vi "Generate Custom Trace.vi"(8 "error in (no error)":errorcluster, 10 "Custom Action":string) -> ()   [LabVIEW 2020, in "Actor Framework.lvlib"]
doc: "<p>Generates a DETT (Desktop Execution Trace Toolkit) User Generated Trace. The trace includes the source actor's ID (or debug alias, if available) and a custom message you define.</p>"
uses:
  Actor Framework.lvlib
  Support/Registration Mode.ctl
  Support/TDM Registration Mode.ctl
  Support/Localized Strings.vi
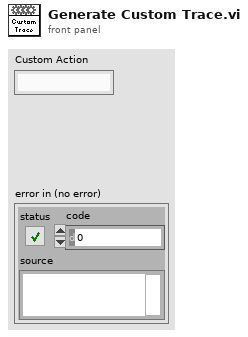
[diagram p1: front panel]
types:
  T1 = typedef "Actor Framework.lvlib/Registration Mode.ctl" = enum16{"Register Actor", "Get ID", "Get Enqueuer", "Deregister Actor", "Get Update Event", "Get All Actors"}
  T2 = typedef "Actor Framework.lvlib/TDM Registration Mode.ctl" = enum16{"Register TDM", "Get ID", "Get Notifier", "Deregister TDM"}
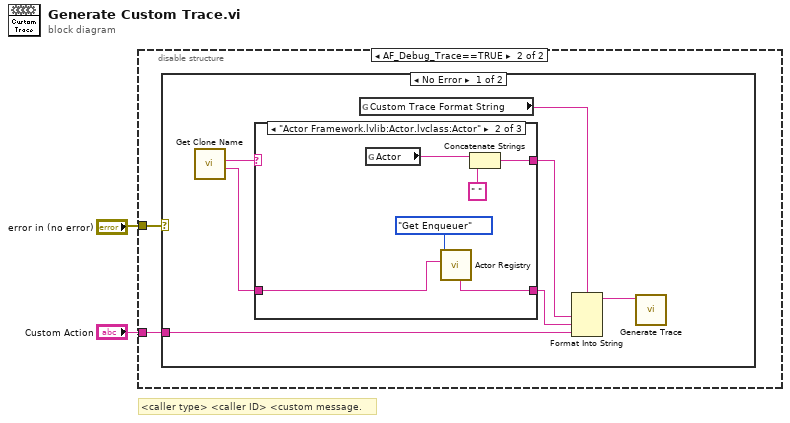
[diagram p0: block diagram]
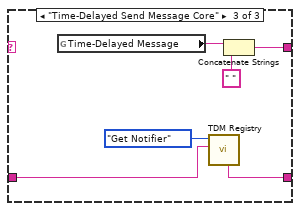
[diagram p4: hidden frame]
diagram:
  # "<caller type> <caller ID> <custom message."
  n1 = disable-structure shown="AF_Debug_Trace==TRUE" {
    disable-tunnel: "Custom Action" -> [_ w4]
    disable-tunnel: "error in (no error)" -> [_ w3]
    frame condition #0 {
    }
    frame condition #1 (active) {
      n2 = case shown="No Error" w3 {
        tunnel: w4 -> [w10 _]
        frame No Error {
          n3 = call "Get Clone Name.vi"() -> ("Clone ID"=w5:string, "Clone Type"=w8:string)  [unwired: 10 in]
          n4 = case shown="\"Actor Framework.lvlib:Actor.lvclass:Actor\"" w8 {
            selector: w8 -> [w13 _ _]
            tunnel: [w13 w19 w25] -> w9
            tunnel: [w12 w15 w21] -> w6
            tunnel: w5 -> [w12 w14 w20]
            frame Default {
            }
            frame "Actor Framework.lvlib:Actor.lvclass:Actor" {
              n5 = global read "Localized Strings.vi" "Actor"() -> (w17:string)
              n6 = call "Actor Registry.vi"("Actor ID"=w14, "Action"=Registration_Mode."Get Enqueuer") -> ("Actor Alias out"=w15:string)  [unwired: 5 in, 4 out]
              n7 = Concatenate Strings(w17, " " ("string")) -> (w19:string)
            }
            frame "Time-Delayed Send Message Core" {
              n8 = global read "Localized Strings.vi" "Time-Delayed Message"() -> (w23:string)
              n9 = call "TDM Registry.vi"("TDM ID"=w20, "Action"=TDM_Registration_Mode."Get Notifier") -> ("TDM Alias Out"=w21:string)  [unwired: 5 in, 4 out]
              n10 = Concatenate Strings(w23, " " ("string")) -> (w25:string)
            }
          }
          n11 = global read "Localized Strings.vi" "Custom Trace Format String"() -> (w7:string)
          n12 = Format Into String(format string=w7, w9, w6, w10) -> (resulting string=w11:string)  [unwired: 2 in, 1 out]
          n13 = call "Generate Trace.vi"("String"=w11) -> ()  [unwired: 11 in]
        }
        frame Error {
        }
      }
    }
  }
